vi "Find All Tests in Directory.vi"(8 "error in (no error)":errorcluster, 10 "Directory Path":path, 11 "LUnit Test Suite In":refnum<class "LUnit Test Suite.lvclass">) -> (0 "error out":errorcluster, 3 "LUnit Test Suite out":refnum<class "LUnit Test Suite.lvclass">)   [LabVIEW 2020, in "Test Finder.lvclass"]
uses:
  Test Finder.lvclass
  LUnit Test Suite.lvclass
  C:/git/astemes-lunit/source/Runnable.lvclass
  <vilib>/Utility/LVClass/Get LV Class Default Value.vi
  LUnit Test Case.lvclass
  Test Finder.lvclass/Test Finder.ctl
  C:/git/astemes-lunit/source/LUnit Test Suite.lvclass
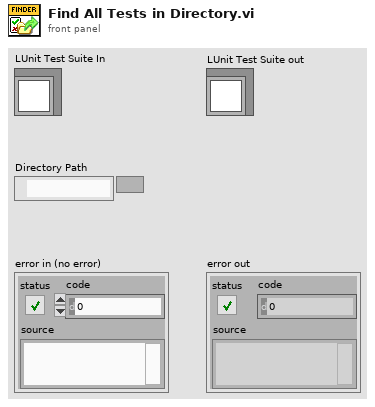
[diagram p1: front panel]
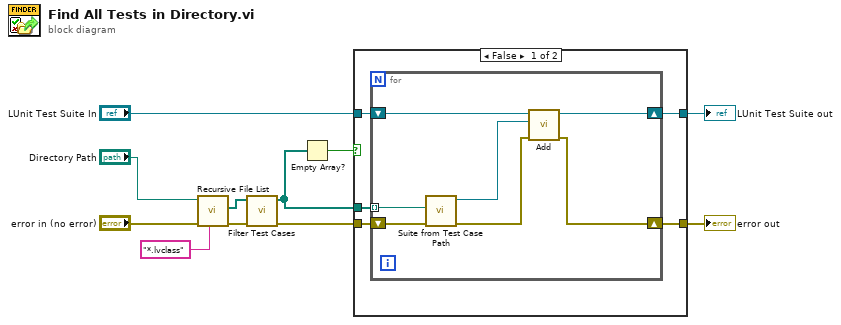
[diagram p0: block diagram]
diagram:
  n1 = call <vilib>:"Recursive File List.vi"("pattern"="*.lvclass", "error in (no error)"="error in (no error)", "Folder Path"="Directory Path") -> ("error out"=w4:errorcluster, "All Files in Dir"=w5:path[])  [unwired: 4 in, 3 out]
  n2 = call "Filter Test Cases.vi"("error in (no error)"=w4, "Classes to Filter"=w5) -> ("error out"=w3:errorcluster, "Filtered Classes"=w2:path[])  [unwired: 8 in]
  n3 = Empty Array?(array=w2) -> (empty?=w1:bool)
  n4 = case shown="False" w1 {
    tunnel: [w16 w25] -> w11
    tunnel: "LUnit Test Suite In" -> [w15 w25]
    tunnel: [w14 w24] -> w9
    tunnel: w3 -> [w13 w24]
    tunnel: w2 -> [w12 _]
    frame False {
      n5 = for {
        shift-right: [w23] -> w16
        shift-left: w15 -> [w22]
        shift-right: [w21] -> w14
        shift-left: w13 -> [w20]
        tunnel: w12 -> [w18] mode=indexing
        n6 = call "Suite from Test Case Path.vi"("error in (no error)"=w20, "Test Case"=w18) -> ("error out"=w19:errorcluster, "LUnit Test Suite Out"=w17:refnum<class "LUnit Test Suite.lvclass">)  [unwired: 8 in]
        n7 = call "Add.vi"("error in (no error)"=w19, "Runnable"=w17, "LUnit Test Suite In"=w22) -> ("error out"=w21:errorcluster, "LUnit Test Suite Out"=w23:refnum<class "LUnit Test Suite.lvclass">)  [unwired: 7 in]
      }
    }
    frame True {
    }
  }
  "LUnit Test Suite out" <- w11
  "error out" <- w9
